vi "Distribution.vi"(0 "Detected Event IN":cluster{dbl[][]}[](array[cluster]), 1 "Sweep trace (2D) In":cluster{"Ramp Pattern":dbl[], "X":dbl[]}[][](array[cluster]), 2 "Threshold":dbl, 3 "Baseline info IN":cluster{dbl[][]}[](array[cluster])) -> (4 "Baseline info new OUT":cluster{dbl[][]}[](array[cluster]), 5 "Averaged amplitude (pA)":dbl[](array[numeric]), 6 "Distribution (output)":T1, 7 "Detected Event (1D) OUT":cluster{dbl[][]}[](array[cluster]), 8 "Sweep trace (2D) Out":cluster{"Ramp Pattern":dbl[], "X":dbl[]}[][](array[cluster]), 9 "Event final OUT":dbl[][](array[numeric]))   [LabVIEW 2017]
uses:
  <vilib>/Analysis/NI_AALPro.lvlib
  <vilib>/Analysis/NI_AALBase.lvlib
panel:
  out "크기":bool
  out "순서":bool
  in  "정지":bool
  out "event":cluster{dbl[], dbl[]}[](graph)
  in  "Event #":i16=4
  in  "Sweep #":i16=4
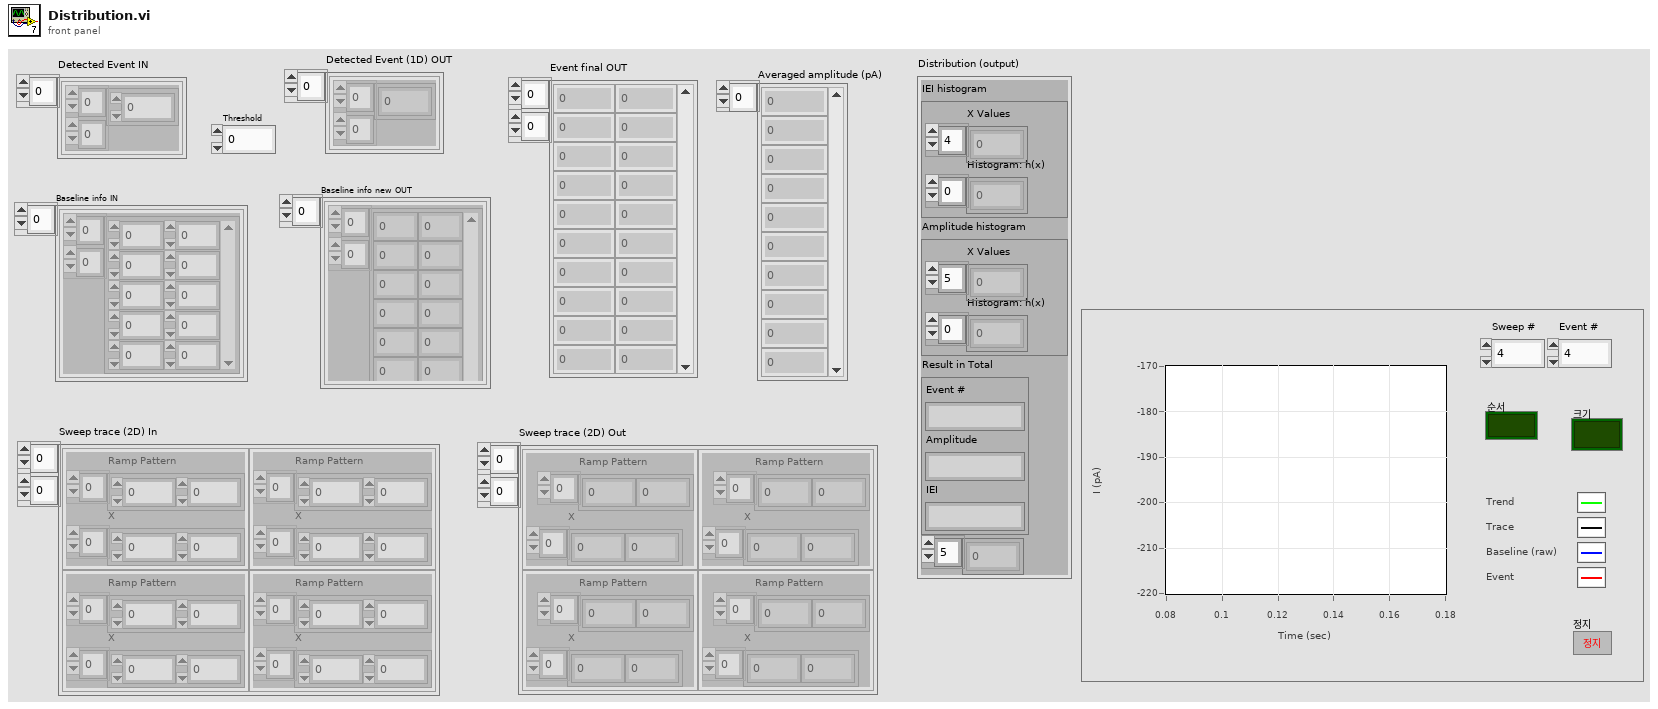
[diagram p1: front panel]
types:
  T1 = cluster{"IEI histogram":cluster{"X Values":dbl[], "Histogram: h(x)":i32[]}, "Amplitude histogram":cluster{"X Values":dbl[], "Histogram: h(x)":i32[]}, "Result in Total ":cluster{"Event #":string, "Amplitude ":string, "IEI":string}, i32[]}
  T2 = cluster{string, "standard deviation":string, "standard deviation":string}
  T3 = cluster{"X Values":dbl[], "Histogram: h(x)":i32[]}
  T4 = cluster{"Histogram Graph":cluster{"X Values":dbl[], "Histogram: h(x)":i32[]}, "Histogram Graph":cluster{"X Values":dbl[], "Histogram: h(x)":i32[]}, cluster{string, "standard deviation":string, "standard deviation":string}, i32[]}
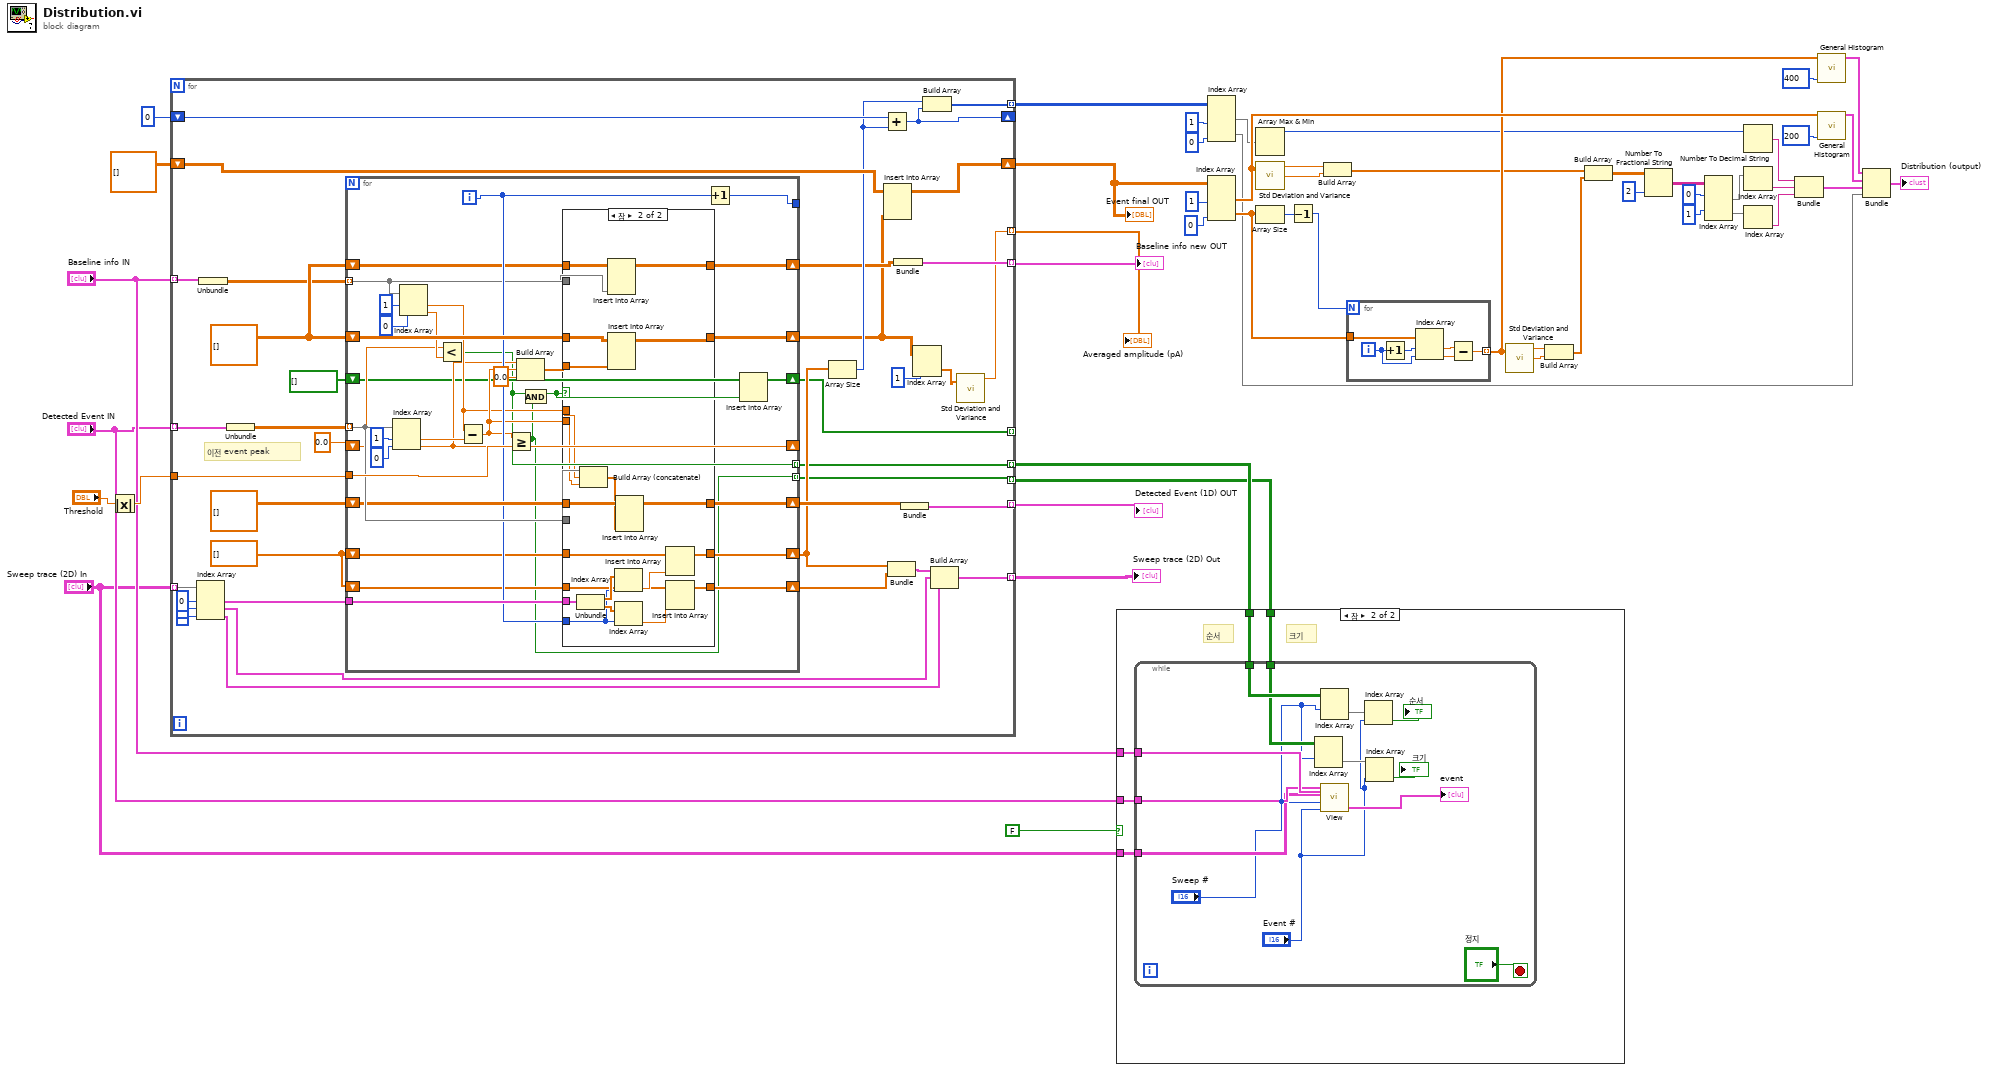
[diagram p0: block diagram]
diagram:
  n1 = Absolute Value(x="Threshold") -> (abs(x)=w11:dbl)
  n2 = for {
    tunnel: "Detected Event IN" -> [w88] mode=indexing
    shift-right: [w58] -> w43
    shift-left: dbl[][] [] -> [w86]
    shift-right: [w84] -> _
    shift-left: 0 ("인덱스") -> [w85]
    tunnel: [w83] -> w30 mode=indexing
    tunnel: w11 -> [w82]
    tunnel: [w79] -> w8 mode=indexing
    tunnel: "Sweep trace (2D) In" -> [w78] mode=indexing
    tunnel: [w68] -> w9 mode=indexing
    tunnel: "Baseline info IN" -> [w66] mode=indexing
    tunnel: [w63] -> w7 mode=indexing
    tunnel: [w59] -> w10 mode=indexing
    tunnel: [w54] -> _ mode=indexing
    tunnel: [w52] -> w3 mode=indexing
    tunnel: [w51] -> w2 mode=indexing
    w75 = dbl[] []
    w65 = dbl[][] []
    # "이전 event peak"
    n3 = Index Array(array=w78, index #1=0 ("인덱스"), index #2=1 ("인덱스"), index #3=2 ("인덱스")) -> (element #1=w76:cluster{"Ramp Pattern":dbl[], "X":dbl[]}, element #2=w70:cluster{"Ramp Pattern":dbl[], "X":dbl[]}, element #3=w69:cluster{"Ramp Pattern":dbl[], "X":dbl[]})
    n4 = Unbundle(w66) -> (w53:dbl[][])
    n5 = Unbundle(w88) -> (w87:dbl[][])
    n6 = for {
      tunnel: w87 -> [w113] mode=indexing
      tunnel: [w115] -> _
      shift-right: [w117] -> w57
      shift-left: w65 -> [w116]
      tunnel: w82 -> [w114]
      shift-right: [w112] -> w80
      shift-left: dbl[][] [] -> [w111]
      tunnel: w76 -> [w109]
      shift-right: [w106] -> w62
      shift-left: w75 -> [w105]
      shift-right: [w107] -> w74
      shift-left: w75 -> [w104]
      tunnel: w53 -> [w101] mode=indexing
      shift-right: [w103] -> w64
      shift-left: w65 -> [w102]
      shift-right: [w96] -> _
      shift-left: 0.0 ("Numeric") -> [w94]
      shift-right: [w92] -> w54
      shift-left: bool[] [] -> [w91]
      tunnel: [w90] -> w52 mode=indexing
      tunnel: [w89] -> w51 mode=indexing
      i -> [w108]
      n7 = Index Array(array=w113, index #1=1 ("인덱스"), index #2=0 ("인덱스")) -> (element #1=w120:dbl, element #2=w96:dbl)
      n8 = Index Array(array=w101, index #1=1 ("인덱스"), index #2=0 ("인덱스")) -> (element #1=w98:dbl, element #2=w95:dbl)
      n9 = Less?(x=w94, y=w95) -> (x < y?=w90:bool)
      n10 = Subtract(x=w98, y=w120) -> (x-y=w99:dbl)
      n11 = Greater Or Equal?(x=w99, y=w114) -> (x >= y?=w89:bool)
      n12 = Build Array(w96, w99, 0.0 ("원소")) -> (w118:dbl[])
      n13 = And(x=w90, y=w89) -> (x .and. y?=w93:bool)
      n14 = case shown="참" w93 {
        tunnel: w118 -> [_ w148]
        tunnel: [w126 w147] -> w117
        tunnel: w116 -> [w126 w146]
        tunnel: w113 -> [_ w130]
        tunnel: [w125 w145] -> w112
        tunnel: w111 -> [w125 w144]
        tunnel: w109 -> [_ w143]
        tunnel: w108 -> [_ w140]
        tunnel: [w123 w137] -> w107
        tunnel: [w124 w136] -> w106
        tunnel: w105 -> [w124 w135]
        tunnel: w104 -> [w123 w134]
        tunnel: w101 -> [_ w133]
        tunnel: [w122 w132] -> w103
        tunnel: w102 -> [w122 w131]
        tunnel: w99 -> [_ w128]
        tunnel: w98 -> [_ w129]
        frame False {
        }
        frame True {
          n15 = Unbundle(w143) -> ("Ramp Pattern"=w142:dbl[], "X"=w141:dbl[])
          n16 = Build Array (concatenate)(w130, w129, w128) -> (w127:dbl[])
          n17 = Insert Into Array(array=w131, new element=w133) -> (w132:dbl[][])  [unwired: 2 in]
          n18 = Insert Into Array(array=w146, new element=w148) -> (w147:dbl[][])  [unwired: 2 in]
          n19 = Index Array(array=w142, index=w140) -> (element=w139:dbl)
          n20 = Index Array(array=w141, index=w140) -> (element=w138:dbl)
          n21 = Insert Into Array(array=w144, new element=w127) -> (w145:dbl[][])  [unwired: 2 in]
          n22 = Insert Into Array(array=w135, new element=w139) -> (w136:dbl[])  [unwired: 1 in]
          n23 = Insert Into Array(array=w134, new element=w138) -> (w137:dbl[])  [unwired: 1 in]
        }
      }
      n24 = Increment(x=w108) -> (x+1=w115:i32)
      n25 = Insert Into Array(array=w91, new element=w93) -> (w92:bool[])  [unwired: 1 in]
    }
    n26 = Array Size(array=w62) -> (size(s)=w67:i32)
    n27 = Add(x=w85, y=w67) -> (x+y=w84:i32)
    n28 = Insert Into Array(array=w86, new element=w57) -> (w58:dbl[][])  [unwired: 2 in]
    n29 = Bundle(w62, w74) -> (w73:cluster{dbl[], dbl[]})  [unwired: 1 in]
    n30 = Bundle(w64) -> (w63:cluster{dbl[][]})  [unwired: 1 in]
    n31 = Bundle(w80) -> (w79:cluster{dbl[][]})  [unwired: 1 in]
    n32 = Index Array(array=w57, index (col)=1 ("비활성화된 인덱스 (열)")) -> (element=w60:dbl[])  [unwired: 1 in]
    n33 = Build Array(w67, w84) -> (w83:i32[])
    n34 = Build Array(w73, w70, w69) -> (w68:cluster{"Ramp Pattern":dbl[], "X":dbl[]}[])
    n35 = call <vilib>:"Std Deviation and Variance.vi"("X"=w60) -> ("mean"=w59:dbl)  [unwired: 1 in, 2 out]
  }
  "Event final OUT" <- w43
  "Detected Event (1D) OUT" <- w8
  "Sweep trace (2D) Out" <- w9
  "Baseline info new OUT" <- w7
  "Averaged amplitude (pA)" <- w10
  n36 = case shown="참" FALSE {
    tunnel: "Baseline info IN" -> [_ w153]
    tunnel: "Detected Event IN" -> [_ w152]
    tunnel: "Sweep trace (2D) In" -> [_ w151]
    tunnel: w3 -> [_ w150]
    tunnel: w2 -> [_ w149]
    frame False {
    }
    frame True {
      # "크기"
      # "순서"
      n37 = while {
        tunnel: w153 -> [w166]
        tunnel: w152 -> [w165]
        tunnel: w151 -> [w164]
        tunnel: w150 -> [w161]
        tunnel: w149 -> [w160]
        stop <- "정지" stop-if-true
        n38 = Index Array(array=w160, index (row)="Sweep #") -> (element=w157:bool[])  [unwired: 1 in]
        n39 = Index Array(array=w161, index (row)="Sweep #") -> (element=w158:bool[])  [unwired: 1 in]
        n40 = call "View.vi"("Event #"="Event #", "Sweep #"="Sweep #", "Baseline info new OUT"=w166, "Sweep trace (2D) In"=w164, "Detected Event (1D) In"=w165) -> ("event"=→"event":cluster{dbl[], dbl[]}[])  [unwired: 3 in, 2 out]
        n41 = Index Array(array=w158, index="Event #") -> (element=→"순서":bool)
        n42 = Index Array(array=w157, index="Event #") -> (element=→"크기":bool)
      }
    }
  }
  n43 = Index Array(array=w30, index (col) #1=1 ("비활성화된 인덱스 (열)"), index (col) #2=0 ("인덱스 (열)")) -> (element #1=w29:i32[], element #2=w14:i32[])  [unwired: 2 in]
  n44 = Index Array(array=w43, index (col) #1=1 ("비활성화된 인덱스 (열)"), index (col) #2=0 ("인덱스 (열)")) -> (element #1=w42:dbl[], element #2=w33:dbl[])  [unwired: 2 in]
  n45 = Array Max & Min(array=w29) -> (max value=w28:i32)  [unwired: 3 out]
  n46 = call <vilib>:"Std Deviation and Variance.vi"("X"=w42) -> ("mean"=w40:dbl, "standard deviation"=w39:dbl)  [unwired: 1 in, 1 out]
  n47 = Array Size(array=w33) -> (size(s)=w48:i32)
  n48 = Decrement(x=w48) -> (x-1=w47:i32)
  n49 = Build Array(w40, w39) -> (w35:dbl[])
  n50 = for {
    N: w47 -> [_]
    tunnel: w33 -> [w172]
    tunnel: [w167] -> w41 mode=indexing
    i -> [w170]
    n51 = Increment(x=w170) -> (x+1=w171:i32)
    n52 = Index Array(array=w172, index #1=w171, index #2=w170) -> (element #1=w169:dbl, element #2=w168:dbl)
    n53 = Subtract(x=w169, y=w168) -> (x-y=w167:dbl)
  }
  n54 = call <vilib>:"Std Deviation and Variance.vi"("X"=w41) -> ("mean"=w37:dbl, "standard deviation"=w38:dbl)  [unwired: 1 in, 1 out]
  n55 = Build Array(w37, w38) -> (w36:dbl[])
  n56 = Build Array(w35, w36) -> (w27:dbl[][])
  n57 = Number To Fractional String(number=w27, precision (6)=i16 2 ("폭(-)")) -> (F-format string=w25:string[][])  [unwired: 2 in]
  n58 = Index Array(array=w25, index (row) #1=0 ("인덱스 (행)"), index (row) #2=1 ("인덱스 (행)")) -> (element #1=w22:string[], element #2=w21:string[])  [unwired: 2 in]
  n59 = Number To Decimal String(number=w28) -> (decimal integer string=w20:string)  [unwired: 1 in]
  n60 = Index Array(array=w22) -> (element=w19:string)  [unwired: 1 in]
  n61 = Index Array(array=w21) -> (element=w18:string)  [unwired: 1 in]
  n62 = Bundle(w20, "standard deviation"=w19, "standard deviation"=w18) -> (w15:T2)  [unwired: 1 in]
  n63 = call <vilib>:"General Histogram.vi"("X"=w41, "# bins"=400) -> ("Histogram Graph"=w17:T3)  [unwired: 9 in, 4 out]
  n64 = call <vilib>:"General Histogram.vi"("X"=w42, "# bins"=200) -> ("Histogram Graph"=w16:T3)  [unwired: 9 in, 4 out]
  n65 = Bundle("Histogram Graph"=w17, "Histogram Graph"=w16, w15, w14) -> (→"Distribution (output)":T4)  [unwired: 1 in]
